vi "Mcp2210 Get Manufacturer String.vi"(8 "error in (no error)":errorcluster, 11 "handle":i32) -> (0 "error out":errorcluster, 2 "Manufacturer":string, 3 "handle out":i32)   [LabVIEW 2015, in "mcp2210.lvlib"]
doc: "Read from device the USB Manufacturer string.\nIn case of successful execution, the function returns 0 (E_SUCCESS) and updates the manufacturerStr\nbuffer.\nIn case of failure, negative error code is returned.\nIf the NVARM string descriptor is invalid, the function returns E_ERR_DESCRIPTOR (-400) error code.\nThe string descriptor is invalid if the String Descriptor ID is not 0x03 or the descriptor size\nis less than 2 or larger than 60 bytes.\nParameters:\nInputs:\n- void *handle - The pointer to the USB device handle. Cannot be NULL.\nOutputs:\n- wchar_t *manufacturerStr - pointer to UNICODE string buffer. Cannot be NULL.\n!! Important details !!\n- the string is NULL (\\0) terminated\n- maximum string length is 29 UNICODE characters =>\nbuffer size must be 60 bytes.\nReturns:\n- 0 for success: E_SUCCESS\n- negative error code: E_ERR_NULL, E_ERR_INVALID_HANDLE_VALUE\nE_ERR_HID_TIMEOUT, E_ERR_HID_RW_FILEIO, E_ERR_UNKOWN_ERROR\nE_ERR_CMD_ECHO, E_ERR_CMD_FAILED\nE_ERR_STRING_DESCRIPTOR\n\nMCP2210_DLL_UM_API int __stdcall Mcp2210_GetManufacturerString(void *handle, unsigned short *manufacturerStr);"
uses:
  <userlib>/mcp2210/mcp2210.lvlib
  <userlib>/mcp2210/mcp2210_dll_um_x86.dll
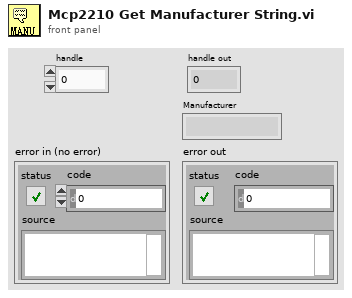
[diagram p1: front panel]
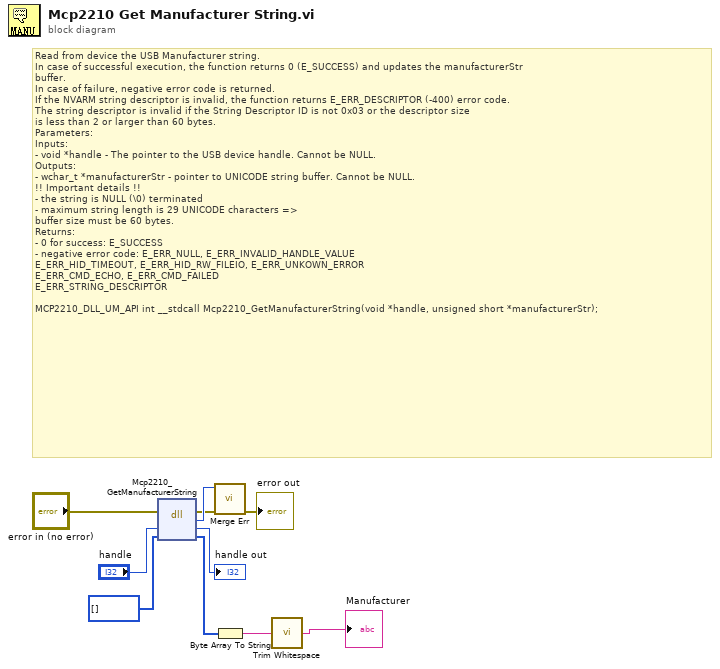
[diagram p0: block diagram]
diagram:
  # "Read from device the USB Manufacturer string.\nIn case of successful execution, the function returns 0 (E_SUCCESS) and updates the manufacturerStr\nbuffer.\nIn case of failure, negative error code is returned.\nIf the NVARM string descriptor is invalid, the function returns E_ERR_DESCRIPTOR (-400) error code.\nThe string descriptor is invalid if the String Descriptor ID is not 0x03 or the descriptor size\nis less than 2 or larger than 60 bytes.\nParameters:\nInputs:\n- void *handle - The pointer to the USB device handle. Cannot be NULL.\nOutputs:\n- wchar_t *manufacturerStr - pointer to UNICODE string buffer. Cannot be NULL.\n!! Important details !!\n- the string is NULL (\\0) terminated\n- maximum string length is 29 UNICODE characters =>\nbuffer size must be 60 bytes.\nReturns:\n- 0 for success: E_SUCCESS\n- negative error code: E_ERR_NULL, E_ERR_INVALID_HANDLE_VALUE\nE_ERR_HID_TIMEOUT, E_ERR_HID_RW_FILEIO, E_ERR_UNKOWN_ERROR\nE_ERR_CMD_ECHO, E_ERR_CMD_FAILED\nE_ERR_STRING_DESCRIPTOR\n\nMCP2210_DLL_UM_API int __stdcall Mcp2210_GetManufacturerString(void *handle, unsigned short *manufacturerStr);"
  n1 = dll-call lib="D:/LabVIEW 2015/user.lib/mcp2210/mcp2210_dll_um_x86.*" fn="Mcp2210_GetManufacturerString"(error in="error in (no error)", "handle"="handle", "manufacturerStr"=u16[] []) -> (error out=w4:errorcluster, "return type"=w5:i32, "handle"=→"handle out":i32, "manufacturerStr"=w7:u16[])  [unwired: 2 in, 1 out]
  n2 = call <userlib>:"Merge Err.vi"("error in (no error)"=w4, "return type"=w5) -> ("error out"=→"error out":errorcluster)  [unwired: 9 in]
  n3 = Byte Array To String(unsigned byte array=w7) -> (string=w6:string)
  n4 = call <vilib>:"Trim Whitespace.vi"("string"=w6) -> ("trimmed string"=→"Manufacturer":string)  [unwired: 1 in]
